vi "SMTP Email No Time Out Error.vi"(7 "error in (no error)":errorcluster) -> (8 "error out":errorcluster)   [LabVIEW 2011, in "NewNI_SMTPEmail.lvlib"]
doc: "No Time Out Error.vi checks if a connection timed out error occurred and resets it to no error."
uses:
  NewNI_SMTPEmail.lvlib
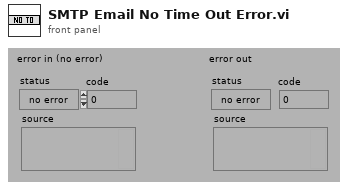
[diagram p1: front panel]
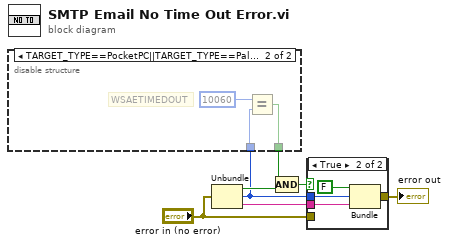
[diagram p0: block diagram]
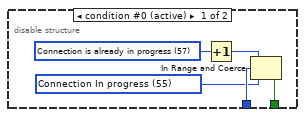
[diagram p2: hidden frame]
diagram:
  n1 = Unbundle("error in (no error)") -> ("status"=w7:bool, "code"=w2:i32, "source"=w3:string)
  n2 = disable-structure shown="TARGET_TYPE==PocketPC||TARGET_TYPE==PalmOS" {
    disable-tunnel: w2 -> [w11 w15]
    disable-tunnel: [w10 w13] -> w1
    frame condition #0 (active) {
      w12 = u16 57 items=["No Error", "Argument Error", "Memory Full", "Out of Zone", "End of File", "File Already Open", "Generic File IO Error", "File Not Found", "File Permission Error", "Disk Full", "Duplicate Path", "Too Many Files Open", "Not Enabled", "Resource File Not Found", "Cannot Add Resource", "Resource Not Found", "Image Not Found", "Image Memory Error", "Pen Does Not Exist", "Config Bad Type", "Config Token Not Found", "Config Parse Error", "Config Memory Error", "Bad External Code Format", "Bad External Code Offset", "External Code Not Present", "Null Window", "Destroy Window Mixup", "Null Menu", "Print Aborted", "Bad Print Record", "Print Driver Error", "Windows Error During Print", "Memory Error During Print", "Print Dialog Error", "Generic Print Error", "Invalid Device Refnum", "Device Not Found", "Device Parameter Error", "Device Unit Error", "Can't Open Device", "Device Call Aborted", "Generic Error", "Cancelled By User", "Object ID Too Low", "Object ID Too High", "Object Not In Heap", "Unknown Heap", "Bad DefProc ID", "DefProc Not In Table", "Message Out Of Range", "Null Method", "Unknown Message", "Manager Call Not Supported", "Bad address", "Connection In progress", "Connection timed out", "Connection is already in progress", "Network attribute not supported", "Network error", "Address in use", "System out of memory", "Connection aborted", "Connection refused", "Connection is not connected", "Connection is already connected", "Connection closed", "Initialize error (interapplication manager)", "Bad occurrence", "Wait on unbound occurrence handler", "Occurrence queue overflow", "Bad path", "Semaphore not signaled", "Unrecognized type (interapplication manager)"]
      w8 = u16 55 items=["No Error", "Argument Error", "Memory Full", "Out of Zone", "End of File", "File Already Open", "Generic File IO Error", "File Not Found", "File Permission Error", "Disk Full", "Duplicate Path", "Too Many Files Open", "Not Enabled", "Resource File Not Found", "Cannot Add Resource", "Resource Not Found", "Image Not Found", "Image Memory Error", "Pen Does Not Exist", "Config Bad Type", "Config Token Not Found", "Config Parse Error", "Config Memory Error", "Bad External Code Format", "Bad External Code Offset", "External Code Not Present", "Null Window", "Destroy Window Mixup", "Null Menu", "Print Aborted", "Bad Print Record", "Print Driver Error", "Windows Error During Print", "Memory Error During Print", "Print Dialog Error", "Generic Print Error", "Invalid Device Refnum", "Device Not Found", "Device Parameter Error", "Device Unit Error", "Can't Open Device", "Device Call Aborted", "Generic Error", "Cancelled By User", "Object ID Too Low", "Object ID Too High", "Object Not In Heap", "Unknown Heap", "Bad DefProc ID", "DefProc Not In Table", "Message Out Of Range", "Null Method", "Unknown Message", "Manager Call Not Supported", "Bad address", "Connection In progress", "Connection timed out", "Connection is already in progress", "Network attribute not supported", "Network error", "Address in use", "System out of memory", "Connection aborted", "Connection refused", "Connection is not connected", "Connection is already connected", "Connection closed", "Initialize error (interapplication manager)", "Bad occurrence", "Wait on unbound occurrence handler", "Occurrence queue overflow", "Bad path", "Semaphore not signaled", "Unrecognized type (interapplication manager)"]
      n3 = Increment(x=w12) -> (x+1=w9:u16)
      n4 = In Range and Coerce(upper limit=w9, x=w11, lower limit=w8) -> (In Range?=w10:bool)  [unwired: 1 out]
    }
    frame condition #1 {
      # "WSAETIMEDOUT"
      n5 = Equal?(x=10060, y=w15) -> (x = y?=w13:bool)
    }
  }
  n6 = Compound Arithmetic op=AND(w1, w7) -> (w6:bool)
  n7 = case shown="True" w6 {
    tunnel: "error in (no error)" -> [w16 _]
    tunnel: w2 -> [_ w18]
    tunnel: [w16 w20] -> w4
    tunnel: w3 -> [_ w19]
    frame False {
    }
    frame True {
      n8 = Bundle(FALSE, "code"=w18, "source"=w19) -> (w20:cluster{bool, "code":i32, "source":string})  [unwired: 1 out]
    }
  }
  "error out" <- w4
